vi "Example 1.vi"() -> ()   [LabVIEW 2016]
uses:
  <vilib>/express/express arith-compare/Formula/XNode/ExpressFormulaBlockNode.xnode
panel:
  out "D":dbl
  in  "Y2":dbl
  in  "Y1":dbl
  in  "X2":dbl
  in  "X1":dbl
  # "DISTANCE"
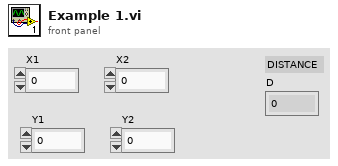
[diagram p1: front panel]
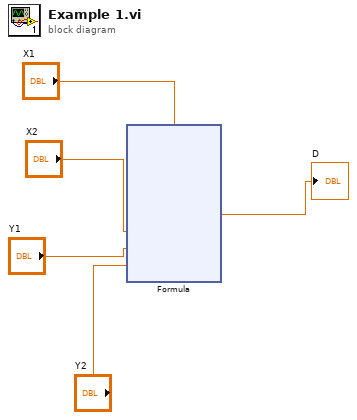
[diagram p0: block diagram]
diagram:
  n1 = xnode "Formula"("X1"="X1", "X2"="X2", "Y1"="Y1", "Y2"="Y2") -> ("Result"=→"D":dbl)  [unwired: 1 in, 1 out]
